vi "Target4.vi"() -> ()   [LabVIEW 2025]
uses:
  <vilib>/Platform/TimedLoop/XDataNode/wakeup.ctl
  <vilib>/Platform/TimedLoop/XDataNode/XDNodeRunTimeDep.lvlib
  <vilib>/Platform/TimedLoop/XDataNode/nitl_modes.ctl
  <vilib>/Platform/TimedLoop/XDataNode/timing_clust.ctl
  <vilib>/platform/TimedLoop/XDataNode/XDataNode.xnode
  <vilib>/rvi/linearAlgebra/MatrixMultiply/XNode/nifxpla_MatrixMultiply.xnode
  <vilib>/rvi/linearAlgebra/MatrixMultiply/simVIs/nifxpla_MatrixMultiply_SimTemplateEinEout.vi
  <vilib>/rvi/linearAlgebra/MatrixMultiply/simVIs/nifxpla_MatrixMultiply_SimTemplateEinVout.vi
  <vilib>/rvi/linearAlgebra/MatrixMultiply/simVIs/nifxpla_MatrixMultiply_SimTemplateVinEout.vi
  <vilib>/rvi/linearAlgebra/MatrixMultiply/simVIs/nifxpla_MatrixMultiply_SimTemplateVinVout.vi
  <vilib>/rvi/DataTransferAndStorage/Container/XNode/niFpgaContainer.xnode
  <vilib>/rvi/interface/RandomDataEmulation/nirviRandomDataFpgaMultiElementTemplate.vi
  <vilib>/rvi/interface/RandomDataEmulation/nirviRandomDataFpgaReadWriteTemplate.vi
panel:
  out "operation overflow":bool
  out "Array 4":fxp<+/-,32,16>[](array[numeric])
  out "Array 5":fxp<+/-,32,16>[](array[numeric])
  out "Array 2":bool[](array[boolean])
  out "Array":bool[](array[boolean])
  out "output valid":bool
  out "Ready for Input":bool
  out "Numeric":i32
  out "Numeric 2":i32
  out "appended array":fxp<+/-,32,16>[](array[numeric])
  out "appended array 2":fxp<+/-,32,16>[](array[numeric])
  out "Array 3":fxp<+/-,32,16>[](array[numeric])
  out "cr":fxp<+/-,32,16>[](array[numeric])
  out "element":fxp<+/-,32,16>
  out "element 2":fxp<+/-,32,16>
  out "ready for a":bool[](array[boolean])
  out "And 1":bool[](array[boolean])
  out "ready for b":bool[](array[boolean])
  out "And 2":bool[](array[boolean])
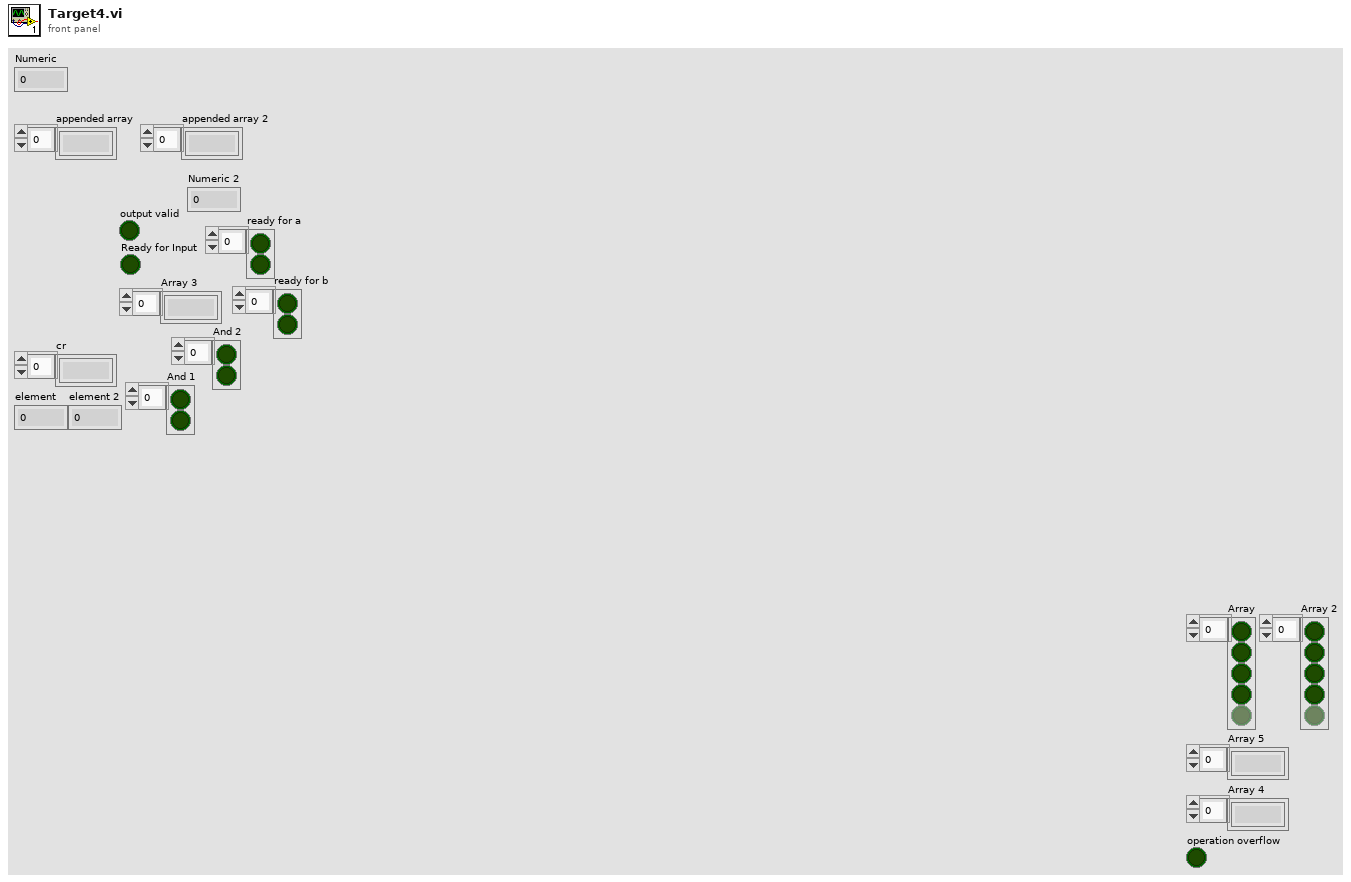
[diagram p1: front panel]
types:
  T1 = typedef "XDNodeRunTimeDep.lvlib/timing_clust.ctl" = cluster{"Expected End [f-1]":u64, "Actual End [f-1]":u64, "Finished Late? [f-1]":bool, "Expected End [i-1]":u64, "Actual End [i-1]":u64, "Finished Late? [i-1]":bool, "Expected Start [i]":u64, "Actual Start [i]":u64, "Expected Start [f]":u64, "Actual Start [f]":u64, "Source Name":string, "Structure Name":string, "Period":i64, "Deadline":i64, "Offset":i64, "Start":i64, "Priority":i32, "Timeout":i32, "Mode":T2, "Wakeup Reason":T3, "Error":errorcluster, "Source Type":string, "Secondary Source Type":string, "Global End Time":u64, "Global Start Time":u64, "Frame Duration":u64, "Iteration Duration":u64, "Assigned CPU":i32, "I/O Scan Engine Mode":u32}
  T2 = typedef "XDNodeRunTimeDep.lvlib/nitl_modes.ctl" = enum32{"No Change", "Process missed periods, maintain original phase", "Discard missed periods, maintain original phase", "Process missed periods, ignore original phase", "Discard missed periods, ignore original phase"}
  T3 = typedef "XDNodeRunTimeDep.lvlib/wakeup.ctl" = enum32{"Normal", "Aborted", "Asynchronous wakeup", "Timing source error", "Timed loop error", "Timeout"}
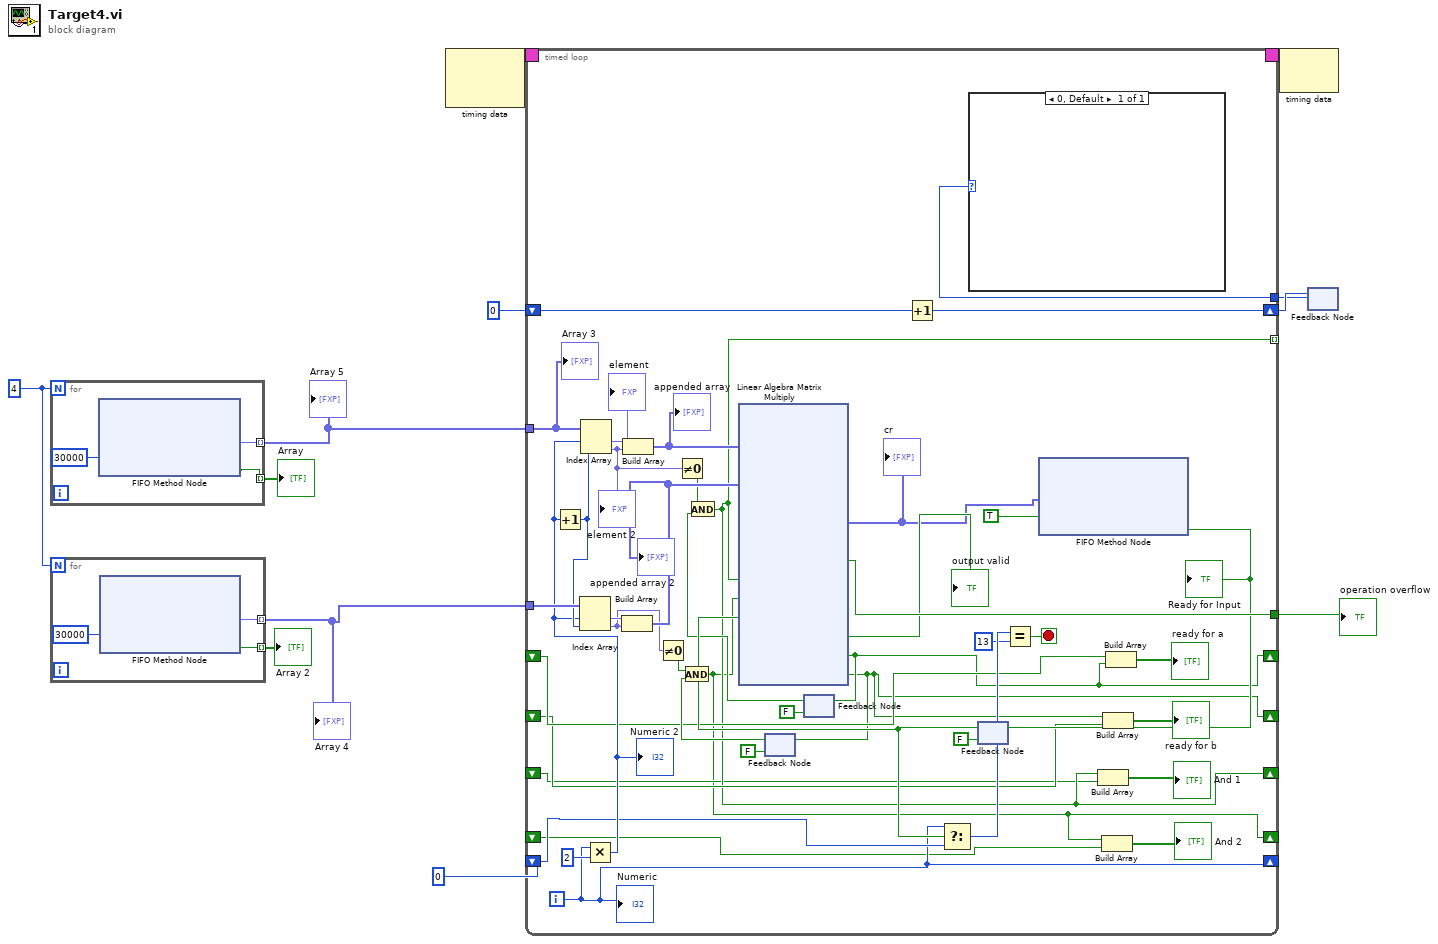
[diagram p0: block diagram]
diagram:
  w10 = 4
  n1 = for {
    N: w10 -> [_]
    tunnel: [w15] -> w6 mode=indexing
    tunnel: [w13] -> w9 mode=indexing
    n2 = xnode ("FIFO Method Node")("Timeout"=30000) -> ("Element"=w15:fxp<+/-,32,16>, "Timed Out?"=w13:bool)  [unwired: 1 in, 1 out]
  }
  "Array" <- w9
  "Array 5" <- w6
  n3 = for {
    N: w10 -> [_]
    tunnel: [w18] -> w5 mode=indexing
    tunnel: [w16] -> w8 mode=indexing
    n4 = xnode ("FIFO Method Node")("Timeout"=30000) -> ("Element"=w18:fxp<+/-,32,16>, "Timed Out?"=w16:bool)  [unwired: 1 in, 1 out]
  }
  "Array 2" <- w8
  "Array 4" <- w5
  n5 = node-c288() -> (w12:T1)  [unwired: 2 in]
  n6 = feedback #1() -> (w1:i16)  [unwired: 1 in]
  n7 = timed-loop {
    timing: w12 -> [_]
    timing-out: [_] -> w11
    tunnel: w6 -> [w45]
    tunnel: w5 -> [w60]
    tunnel: [w52] -> w7
    shift-right: [w41] -> _
    shift-left: 0 -> [w42]
    tunnel: [w25] -> _ mode=indexing
    shift-right: [w32] -> _
    shift-left: _ -> [w33]
    shift-right: [w27] -> _
    shift-left: _ -> [w26]
    shift-right: [w25] -> _
    shift-left: _ -> [w24]
    shift-right: [w22] -> _
    shift-left: _ -> [w23]
    shift-right: [w20] -> w2
    shift-left: i16 0 -> [w21]
    tunnel: w1 -> [w19]
    i -> [w41]
    stop <- w56 stop-if-true
    n8 = Multiply(x=w41, y=2) -> (x*y=w43:i32)
    "Numeric 2" <- w43
    n9 = Increment(x=w43) -> (x+1=w49:i32)
    n10 = Index Array(array=w60, index #1=w43, index #2=w49) -> (element #1=w61:fxp<+/-,32,16>, element #2=w39:fxp<+/-,32,16>)
    n11 = Index Array(array=w45, index #1=w43, index #2=w49) -> (element #1=w62:fxp<+/-,32,16>, element #2=w34:fxp<+/-,32,16>)
    "element" <- w62
    "element 2" <- w34
    n12 = Build Array(w61, w39) -> (w40:fxp<+/-,32,16>[])
    "appended array 2" <- w40
    n13 = Build Array(w62, w34) -> (w46:fxp<+/-,32,16>[])
    "appended array" <- w46
    n14 = Not Equal To 0?(x=w39) -> (x != 0?=w38:bool)
    n15 = Not Equal To 0?(x=w34) -> (x != 0?=w36:bool)
    n16 = feedback #2(FALSE ("ready for b")) -> (w37:bool)
    n17 = And(x=w38, y=w37) -> (x .and. y?=w22:bool)
    n18 = feedback #3(FALSE ("ready for a")) -> (w35:bool)
    n19 = And(x=w36, y=w35) -> (x .and. y?=w25:bool)
    n20 = Increment(x=w21) -> (x+1=w20:i16)
    n21 = case shown="0, Default" w19 {
      frame 0, Default {
      }
    }
    n22 = feedback #4(FALSE ("Ready for Input")) -> (w57:bool)
    n23 = xnode ("Linear Algebra Matrix Multiply")("ar"=w46, "br"=w40, "a valid"=w25, "b valid"=w22, "ready for output (T)"=w57) -> ("cr"=w47:fxp<+/-,32,16>[], "operation overflow"=w52:bool, "output valid"=→"output valid":bool, "ready for a"=w32:bool, "ready for b"=w27:bool)  [unwired: 2 in, 1 out]
    "cr" <- w47
    n24 = feedback-in #2(w27) -> ()
    n25 = feedback-in #3(w32) -> ()
    n26 = Select(t=w41, s=w57, f=w42) -> (s? t:f=w55:i32)
    n27 = Equal?(x=w55, y=13) -> (x = y?=w56:bool)
    n28 = xnode ("FIFO Method Node")("Element"=w47, "Input Valid"=TRUE) -> ("Ready for Input"=w51:bool)  [unwired: 1 in, 1 out]
    "Ready for Input" <- w51
    n29 = feedback-in #4(w51) -> ()
    n30 = Build Array(w25, w24) -> (→"And 1":bool[])
    n31 = Build Array(w22, w23) -> (→"And 2":bool[])
    n32 = Build Array(w27, w26) -> (→"ready for b":bool[])
    n33 = Build Array(w33, w32) -> (→"ready for a":bool[])
    "Numeric" <- w41
    "Array 3" <- w45
  }
  "operation overflow" <- w7
  n34 = node-c288(w11) -> ()  [unwired: 1 out]
  n35 = feedback-in #1(w2) -> ()
